vi "VNARP - LAUNCH.vi"(11 "RP IP":string="192.168.0.2") -> (3 "VNA launched ?":bool)   [LabVIEW 2021]
uses:
  Field R&D Services/LIBSSH2 for LabVIEW/Toolkit/Session/Support/Create from SSH.vi
  Field R&D Services/LIBSSH2 for LabVIEW/Toolkit/Session/Support/Password Authentication.vi
  Field R&D Services/LIBSSH2 for LabVIEW/Toolkit/Channel/Support/Create from Session.vi
  Field R&D Services/LIBSSH2 for LabVIEW/Toolkit/Channel/Support/Destroy to Session.vi
  Field R&D Services/LIBSSH2 for LabVIEW/Toolkit/Session/Support/Destroy to SSH.vi
  Field R&D Services/LIBSSH2 for LabVIEW/Toolkit/Session/Session.lvclass
  Field R&D Services/LIBSSH2 for LabVIEW/Toolkit/Channel/Channel.lvclass
  Field R&D Services/LIBSSH2 for LabVIEW/Toolkit/SSH/SSH.lvclass
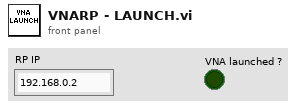
[diagram p1: front panel]
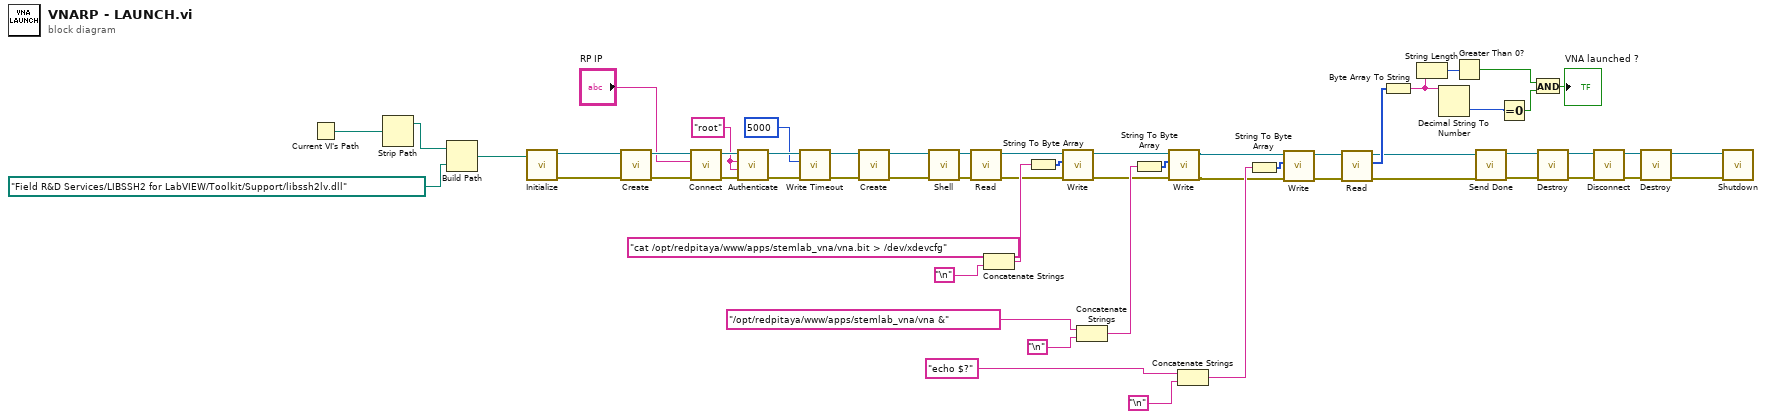
[diagram p0: block diagram]
diagram:
  w51 = "root" ("Username")
  n1 = Current VI's Path() -> (path=w9:path)
  n2 = Strip Path(path=w9) -> (stripped path=w6:path)  [unwired: 1 out]
  n3 = Build Path(base path=w6, name or relative path=path "Field R&D Services/LIBSSH2 for LabVIEW/Toolkit/Support/libssh2lv.dll" ("libssh2lv Shared Library")) -> (appended path=w8:path)
  n4 = call "Initialize.vi"("libssh2lv Shared Library"=w8) -> ("Error Out"=w57:errorcluster, "SSH"=w58:refnum<class "SSH.lvclass">)  [unwired: 9 in]
  n5 = call-poly "Create.vi"("Error In"=w57, "SSH"=w58) -> ("Error Out"=w55:errorcluster, "Sesssion"=w56:refnum<class "Session.lvclass">)  [unwired: 8 in]
  n6 = call "Connect.vi"("Error In"=w55, "Address"="RP IP", "Session In"=w56) -> ("Error Out"=w52:errorcluster, "Sesssion Out"=w53:refnum<class "Session.lvclass">)  [unwired: 7 in]
  n7 = call-poly "Authenticate.vi"("Error In"=w52, "Password"=w51, "Username"=w51, "Session In"=w53) -> ("Error Out"=w42:errorcluster, "Sesssion Out"=w43:refnum<class "Session.lvclass">)  [unwired: 6 in]
  n8 = call "Write Timeout.vi"("Error In"=w42, "Timeout"=5000, "Session In"=w43) -> ("Error Out"=w41:errorcluster, "Sesssion Out"=w40:refnum<class "Session.lvclass">)  [unwired: 7 in]
  n9 = call-poly "Create.vi"("Error In"=w41, "Session"=w40) -> ("Error Out"=w49:errorcluster, "Channel"=w50:refnum<class "Channel.lvclass">)  [unwired: 8 in]
  n10 = call "Shell.vi"("Error In"=w49, "Channel In"=w50) -> ("Error Out"=w44:errorcluster, "Channel Out"=w45:refnum<class "Channel.lvclass">)  [unwired: 8 in]
  n11 = call "Read.vi"("Error In"=w44, "Channel In"=w45) -> ("Error Out"=w24:errorcluster, "Channel Out"=w25:refnum<class "Channel.lvclass">)  [unwired: 7 in, 1 out]
  n12 = Concatenate Strings("cat /opt/redpitaya/www/apps/stemlab_vna/vna.bit > /dev/xdevcfg", "\n") -> (w30:string)
  n13 = String To Byte Array(string=w30) -> (unsigned byte array=w46:u8[])
  n14 = call "Write.vi"("Error In"=w24, "Data"=w46, "Channel In"=w25) -> ("Error Out"=w22:errorcluster, "Channel Out"=w23:refnum<class "Channel.lvclass">)  [unwired: 6 in, 1 out]
  n15 = Concatenate Strings("/opt/redpitaya/www/apps/stemlab_vna/vna &", "\n") -> (w26:string)
  n16 = String To Byte Array(string=w26) -> (unsigned byte array=w29:u8[])
  n17 = call "Write.vi"("Error In"=w22, "Data"=w29, "Channel In"=w23) -> ("Error Out"=w18:errorcluster, "Channel Out"=w19:refnum<class "Channel.lvclass">)  [unwired: 6 in, 1 out]
  n18 = Concatenate Strings("echo $?", "\n") -> (w20:string)
  n19 = String To Byte Array(string=w20) -> (unsigned byte array=w21:u8[])
  n20 = call "Write.vi"("Error In"=w18, "Data"=w21, "Channel In"=w19) -> ("Error Out"=w15:errorcluster, "Channel Out"=w14:refnum<class "Channel.lvclass">)  [unwired: 6 in, 1 out]
  n21 = call "Read.vi"("Error In"=w15, "Channel In"=w14) -> ("Error Out"=w10:errorcluster, "Data"=w13:u8[], "Channel Out"=w11:refnum<class "Channel.lvclass">)  [unwired: 7 in]
  n22 = Byte Array To String(unsigned byte array=w13) -> (string=w5:string)
  n23 = String Length(string=w5) -> (length=w4:i32)
  n24 = Decimal String To Number(string=w5) -> (number=w12:i32)  [unwired: 2 in, 1 out]
  n25 = Greater Than 0?(x=w4) -> (x > 0?=w1:bool)
  n26 = call "Send Done.vi"("Error In"=w10, "Channel In"=w11) -> ("Error Out"=w33:errorcluster, "Channel Out"=w34:refnum<class "Channel.lvclass">)  [unwired: 8 in]
  n27 = Equal To 0?(x=w12) -> (x = 0?=w2:bool)
  n28 = And(x=w1, y=w2) -> (x .and. y?=→"VNA launched ?":bool)
  n29 = call-poly "Destroy.vi"("Error In"=w33, "Channel"=w34) -> ("Error Out"=w36:errorcluster, "Session"=w35:refnum<class "Session.lvclass">)  [unwired: 8 in]
  n30 = call "Disconnect.vi"("Error In"=w36, "Session In"=w35) -> ("Error Out"=w37:errorcluster, "Sesssion Out"=w38:refnum<class "Session.lvclass">)  [unwired: 8 in]
  n31 = call-poly "Destroy.vi"("Error In"=w37, "Session"=w38) -> ("Error Out"=w47:errorcluster, "SSH"=w48:refnum<class "SSH.lvclass">)  [unwired: 8 in]
  n32 = call "Shutdown.vi"("Error In"=w47, "SSH"=w48) -> ()  [unwired: 9 in, 1 out]
